vi "CIMAQ_Skeleton_Branches.vi"(0 "Skeleton in":T1, 1 "Branches dst":T1) -> (5 "Branches":T1)   [LabVIEW 2017]
uses:
  <vilib>/vision/Image Controls.llb/IMAQ Image.ctl
  <vilib>/vision/NI_Vision_Development_Module.lvlib
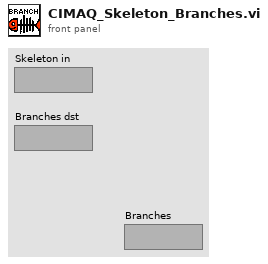
[diagram p1: front panel]
types:
  T1 = typedef "IMAQ Image.ctl" = refnum<image>
  T2 = enum32{"Average", "Min", "Max", "Clear  if < ", "Clear  if < or =", "Clear  if =", "Clear  if > or =", "Clear  if >"}
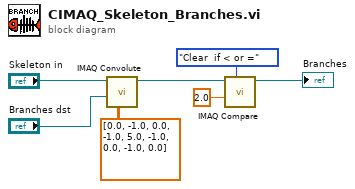
[diagram p0: block diagram]
diagram:
  n1 = call "IMAQ Convolute"("Kernel"=sgl[][] [[0.0, -1.0, 0.0], [-1.0, 5.0, -1.0], [0.0, -1.0, 0.0]], "Image Dst"="Branches dst", "Image Src"="Skeleton in") -> ("Image Dst Out"=w7:T1)  [unwired: 4 in, 4 out]
  n2 = call "IMAQ Compare"("Constant"=sgl 2.0, "Operator"=T2."Clear  if < or =", "Image Src A"=w7) -> ("Image Dst Out"=→"Branches":T1)  [unwired: 7 in, 1 out]
